vi "ReadPicoAmmeter.vi"(8 "error in (no error)":errorcluster, 10 "Connected":bool, 11 "PicoAmmeter":refnum<visa-resource-name>) -> (0 "error out":errorcluster, 2 "Current":dbl)   [LabVIEW 2024]
uses:
  <instrlib>/Keithley 648X Series/Keithley 648X Series.lvlib
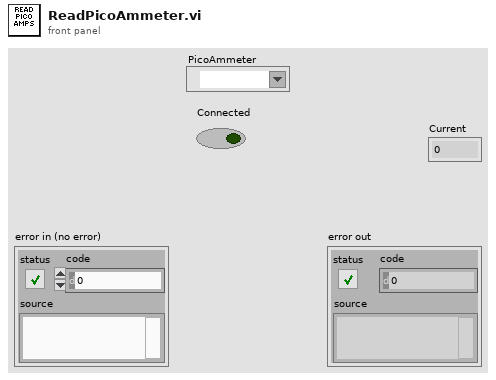
[diagram p1: front panel]
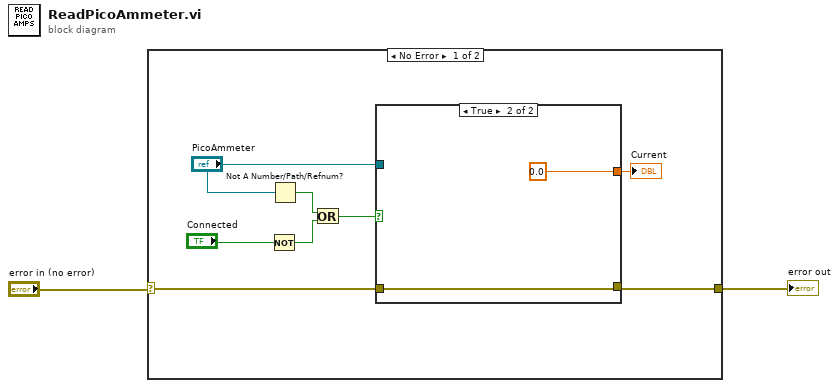
[diagram p0: block diagram]
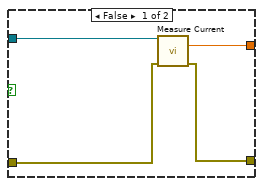
[diagram p2: hidden frame]
diagram:
  n1 = case shown="No Error" "error in (no error)" {
    selector: "error in (no error)" -> [w4 w17]
    tunnel: [w3 w17] -> w1
    frame No Error {
      n2 = Not(x="Connected") -> (.not. x?=w8:bool)
      n3 = Not A Number/Path/Refnum?(number/path/refnum="PicoAmmeter") -> (NaN/Path/Refnum?=w9:bool)
      n4 = Or(x=w9, y=w8) -> (x .or. y?=w7:bool)
      n5 = case shown="True" w7 {
        tunnel: [w14 0.0] -> w5
        tunnel: "PicoAmmeter" -> [w13 _]
        tunnel: w4 -> [w12 w15]
        tunnel: [w11 w15] -> w3
        frame False {
          n6 = call <instrlib>:"Measure Current.vi"("VISA resource name"=w13, "error in (no error)"=w12) -> ("Measurement"=w14:dbl, "error out"=w11:errorcluster)  [unwired: 11 in, 1 out]
        }
        frame True {
        }
      }
      "Current" <- w5
    }
    frame Error {
    }
  }
  "error out" <- w1
